vi "Divide.vi"(10 "x":dbl, 11 "y":dbl) -> (2 "x/y":dbl)   [LabVIEW 2021]
panel:
  out "Graphe":dbl[](graph)
  in  "Booléen":bool
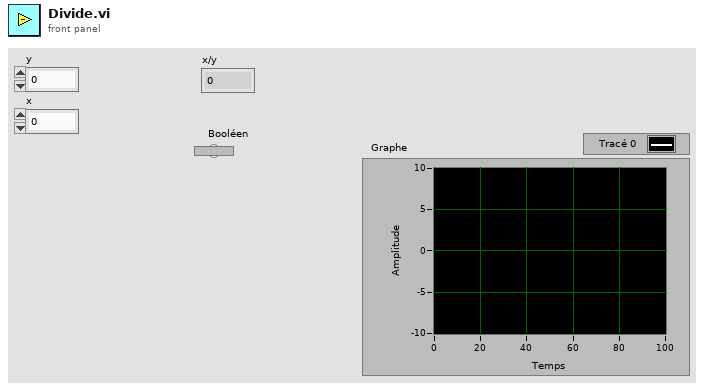
[diagram p1: front panel]
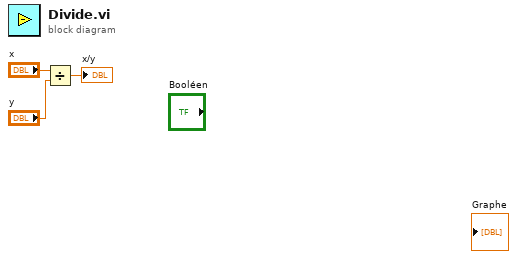
[diagram p0: block diagram]
diagram:
  n1 = Divide(x="x", y="y") -> (x/y=→"x/y":dbl)
